vi "Filter.vi"(2 "on/off":bool, 3 "Cutoff freq (Hz)":dbl, 4 "error in":errorcluster, 5 "signal in":waveform(dbl)={"t0"=timestamp(0 s since 1904-01-01), "dt"=0.001, "Y"=[]}) -> (0 "error out":errorcluster, 1 "signal out":waveform(dbl))   [LabVIEW 2019]
uses:
  <vilib>/measure/macond.llb/FIR Filter for 1 Chan.vi
  <vilib>/measure/NI_MAPro.lvlib
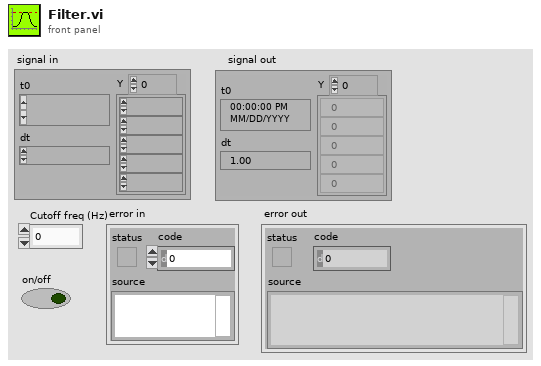
[diagram p1: front panel]
types:
  T1 = cluster{"Topology":enum16{"Off", "FIR by Specification", "Equi-ripple FIR", "Windowed FIR"}, "Type":enum16{"Lowpass", "Highpass", "Bandpass", "Bandstop"}, "#Taps":i32, "Lower PB":dbl, "Upper PB":dbl, "Lower SB":dbl, "Upper SB":dbl}
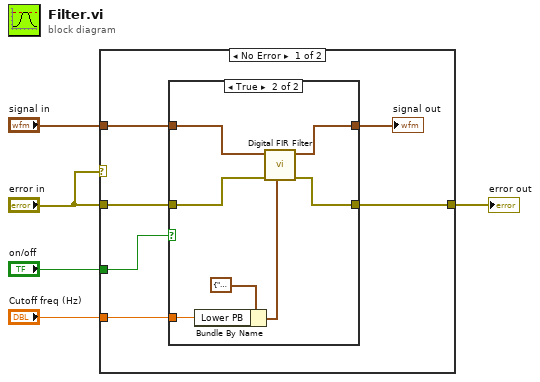
[diagram p0: block diagram]
diagram:
  n1 = case shown="No Error" "error in" {
    tunnel: "error in" -> [w11 w21]
    tunnel: "signal in" -> [w10 _]
    tunnel: [w9 w21] -> w1
    tunnel: "Cutoff freq (Hz)" -> [w8 _]
    tunnel: "on/off" -> [w7 _]
    frame No Error {
      n2 = case shown="True" w7 {
        tunnel: w11 -> [w13 w20]
        tunnel: w10 -> [w12 w19]
        tunnel: [w13 w18] -> w9
        tunnel: w8 -> [_ w17]
        tunnel: [w12 w15] -> w6
        frame False {
        }
        frame True {
          n3 = Bundle By Name(cluster=T1 {"Topology"=enum."Windowed FIR", "Type"=enum."Lowpass", "#Taps"=50, "Lower PB"=100.0, "Upper PB"=0.0, "Lower SB"=200.0, "Upper SB"=0.0} ("FIR filter specifications"), "Lower PB"=w17) -> (w16:T1)
          n4 = call-poly <vilib>:"Digital FIR Filter.vi"("FIR filter specifications"=w16, "error in (no error)"=w20, "signal in"=w19) -> ("error out"=w18:errorcluster, "signal out"=w15:waveform(dbl))  [unwired: 6 in, 1 out]
        }
      }
      "signal out" <- w6
    }
    frame Error {
    }
  }
  "error out" <- w1
